vi "AttackPs.vi"(8 "error in (no error)":errorcluster, 9 "Game in":refnum<class "Game.lvclass">, 10 "Robot":refnum<class "Robot.lvclass">, 11 "AttackPs in":refnum<class "AttackPs.lvclass">) -> (0 "error out":errorcluster, 2 "Robot out":refnum<class "Robot.lvclass">, 3 "AttackPs out":refnum<class "AttackPs.lvclass">)   [LabVIEW 2023, in "AttackPs.lvclass"]
uses:
  AttackPs.lvclass
  Game_class/Game.lvclass
  Robot_class/Robot.lvclass
  Robot_class/Robot.lvclass/Robot.ctl
  Robot_class/Write dest_x.vi
  Robot_class/Write dest_y.vi
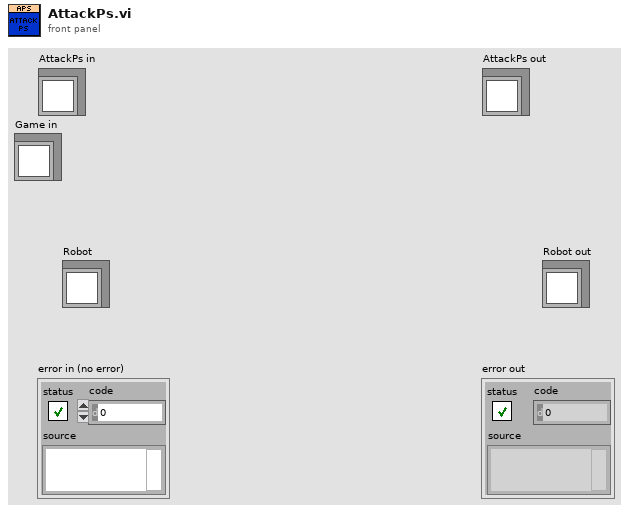
[diagram p1: front panel]
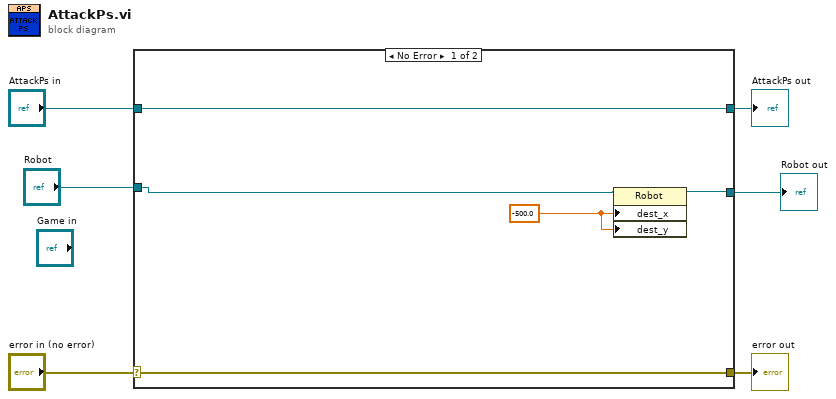
[diagram p0: block diagram]
diagram:
  n1 = case shown="No Error" "error in (no error)" {
    selector: "error in (no error)" -> [w10 w14]
    tunnel: [w10 w14] -> w5
    tunnel: [w11 w13] -> w3
    tunnel: "AttackPs in" -> [w11 w13]
    tunnel: "Robot" -> [w9 w12]
    tunnel: [w8 w12] -> w1
    frame No Error {
      w7 = -500.0 ("dest_x")
      n2 = property class="Robot"(reference=w9, "dest_x"=w7, "dest_y"=w7) -> (reference out=w8:refnum<class "Robot.lvclass">)  [unwired: 1 in, 1 out]
    }
    frame Error {
    }
  }
  "error out" <- w5
  "AttackPs out" <- w3
  "Robot out" <- w1
